vi "State Estimator.vi"(0 "Error In":errorcluster, 1 "State Estimate In":refnum<data-value>, 5 "Matrices":T6={"B"=[0.0, 0.0, 0.0, 0.0, 0.026179, 0.01, 0.0], "A"=[[1.0, 0.0, 0.0, 0.0, 0.0, 0.0, 0.01], [0.0, 1.0, 0.03, 0.0, 0.0, 0.01278, 0.0], [0.0, 0.0, 1.0, 0.0, 0.0, 0.025745, 0.0], [0.0, 0.0, 0.0, 1.0, 0.01, 0.0, 0.0], [0.0, 0.0, 0.0, 0.18884, 1.0, 0.13938, 0.0], [0.0, 0.0, 0.0, 0.0, 0.0, 1.0, 0.0], [0.0, 0.0, 0.0, 0.0, 0.0, 0.0, 1.0]], "C"=[[1.0, 0.0, 0.0, 0.0, 0.0, 0.0, 0.0], [0.0, 1.0, 0.0, 0.0, 0.0, 0.0, 0.0], [0.0, 0.0, 0.0, -13.87, 0.0, 4.7268, 0.0], [0.0, 0.0, 0.0, 0.0, 1.0, 0.0, 0.0], [0.0, 0.0, 0.0, 0.0, 0.0, 2.5745, 0.0], [0.0, 0.0, 0.0, 0.0, 0.0, 1.0, 0.0], [0.0, 0.0, 0.0, 0.0, 0.0, 0.0, 1.0]], "D"=[0.0, 0.0, -0.56285, 0.0, 0.0, 0.0, 0.0], "K"=[[0.61806, 0.0, 0.0, 0.0, 0.0, 0.0, 0.007236], [0.0, 0.64745, 1.9709e-05, 7.2294e-05, 0.0040091, 0.0015572, 0.0], [0.0, 0.60898, 2.0597e-05, 0.00027735, 0.0083707, 0.0032514, 0.0], [0.0, 2.3784e-05, 0.0, 0.0066165, 0.1014, 0.039387, 0.0], [0.0, 6.3434e-05, 0.0, 0.6191, 0.063823, 0.024791, 0.0], [0.0, 6.6011e-05, 0.0025018, 0.0011774, 0.29882, 0.11607, 0.0], [0.0010557, 0.0, 0.0, 0.0, 0.0, 0.0, 0.61803]], "Trajectory"=array601x3[1803 elements], "Init"=[0.0, 0.0, -0.56285, 0.0, 0.0, 0.0, 0.0]}, 7 "Configuration":T1={"Accelerometer Bias"={"X (m/s)"=0.0, "Y (m/s)"=0.0, "Z (m/s)"=0.0}, "Gyroscope Bias"={"X (m/s)"=0.0, "Y (m/s)"=0.0, "Z (m/s)"=0.0}, "Steering Motor Gear Ratio"=611.0, "Steering Pully Gear Ratio"=1.0, "Steering Encoder CPR"=500.0, "Steering Motor Max RPM"=4000.0, "Wheelbase (m)"=1.12, "Fork Angle (rad)"=1.3, "Balancing Controller"={"Kp (/s)"=1.0, "Kd (1)"=1.0}, "Max Allowed Steering Angle (rad)"=0.7, "Task Periods"={"Emergency Stop (us)"=10000, "IMU (us)"=10000, "Steering Motor Encoder (us)"=10000, "State Estimator (us)"=10000, "Balancing Controller (us)"=10000, "GNSS (us)"=10000, "Logging (us)"=50000, "Drive Motor (us)"=100000}, "Drive Motor Gear Ratio"=0.7, "lr"=0.0, "lf"=0.0, "lambda"=0.0, "k1"=0.0, "k2"=0.0, "e1_max"=0.0, "Ad_t"=0.0, "Bd_t"=0.0, "C_t"=0.0, "D_t"=0.0, "Wheel radius"=0.311}, 9 "Iteration":dbl, 11 "Measurement In":refnum<data-value>, 12 "Balancing controller In":refnum<data-value>) -> (4 "Error out":errorcluster, 15 "Measurement Out":refnum<data-value>)   [LabVIEW 2021]
uses:
  Measurements.ctl
  IMU/IMU Data.ctl
  Steering Motor Encoder/Steering Motor Encoder Data.ctl
  GNSS/GNSS Data.ctl
  Logging/Controller Data.ctl
  Drive Motor/Drive Motor Data.ctl
  Steering Motor/Steering Motor Data.ctl
  State Estimate.ctl
  Configuration/Configuration.ctl
panel:
  in  "Byte Stream File Refnum":refnum<file>
  out "Flag GPS":dbl
  out "State Estimate Out":refnum<data-value>
  out "data value":T2
  out "Input measurements":T5
  out "output cluster":T5 {"Y (m)" format="%#_10g"; "X (m)" format="%#_10g"}
  out "Balancing controller Out":refnum<data-value>
  in  "path in":path=path "libkalman_filter.so"
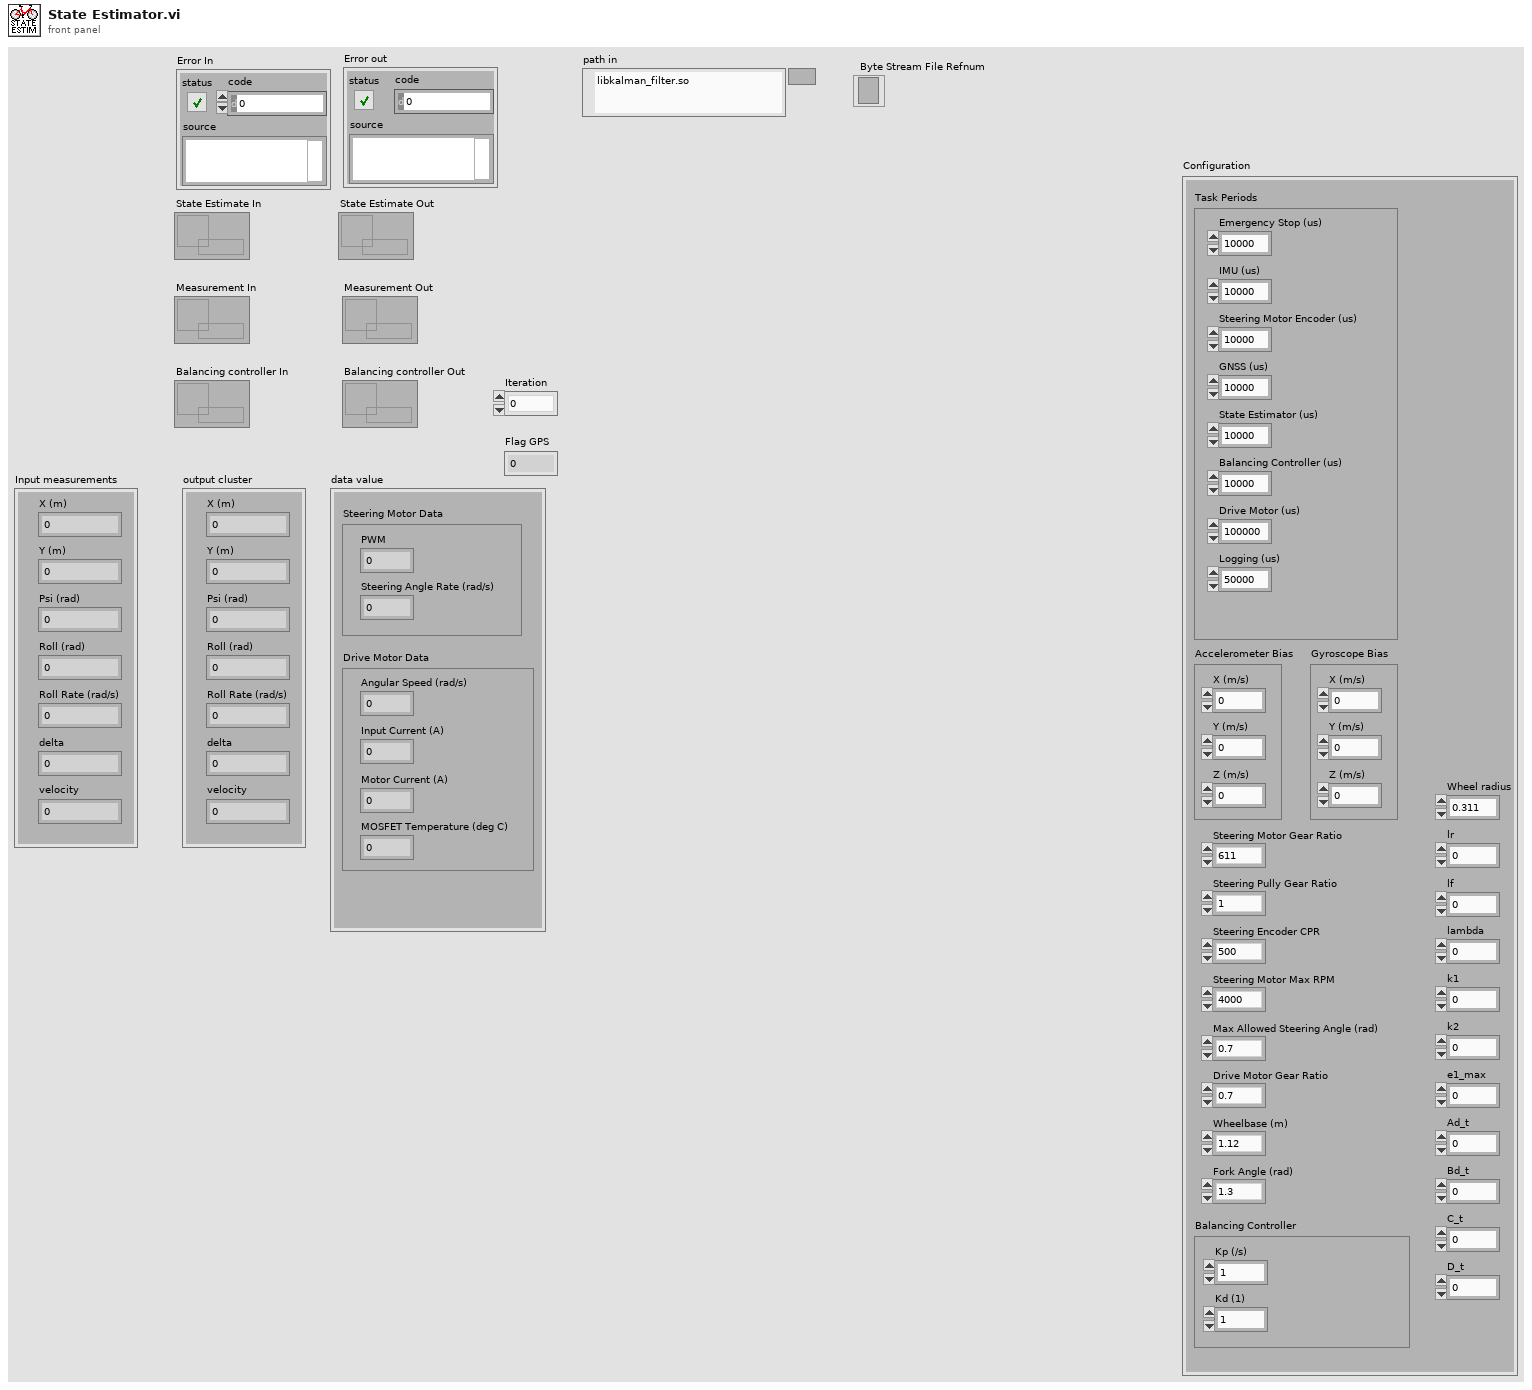
[diagram p1: front panel]
types:
  T1 = typedef "Configuration.ctl" = cluster{"Accelerometer Bias":cluster{"X (m/s)":dbl, "Y (m/s)":dbl, "Z (m/s)":dbl}, "Gyroscope Bias":cluster{"X (m/s)":dbl, "Y (m/s)":dbl, "Z (m/s)":dbl}, "Steering Motor Gear Ratio":dbl, "Steering Pully Gear Ratio":dbl, "Steering Encoder CPR":dbl, "Steering Motor Max RPM":dbl, "Wheelbase (m)":dbl, "Fork Angle (rad)":dbl, "Balancing Controller":cluster{"Kp (/s)":dbl, "Kd (1)":dbl}, "Max Allowed Steering Angle (rad)":dbl, "Task Periods":cluster{"Emergency Stop (us)":i64, "IMU (us)":i64, "Steering Motor Encoder (us)":i64, "State Estimator (us)":i64, "Balancing Controller (us)":i64, "GNSS (us)":i64, "Logging (us)":i64, "Drive Motor (us)":i64}, "Drive Motor Gear Ratio":dbl, "lr":dbl, "lf":dbl, "lambda":dbl, "k1":dbl, "k2":dbl, "e1_max":dbl, "Ad_t":dbl, "Bd_t":dbl, "C_t":dbl, "D_t":dbl, "Wheel radius":dbl}
  T2 = typedef "Controller Data.ctl" = cluster{"Drive Motor Data":T3, "Steering Motor Data":T4}
  T3 = typedef "Drive Motor Data.ctl" = cluster{"Angular Speed (rad/s)":dbl, "Input Current (A)":dbl, "Motor Current (A)":dbl, "MOSFET Temperature (deg C)":dbl}
  T4 = typedef "Steering Motor Data.ctl" = cluster{"PWM":dbl, "Steering Angle Rate (rad/s)":dbl}
  T5 = typedef "State Estimate.ctl" = cluster{"X (m)":dbl, "Y (m)":dbl, "Psi (rad)":dbl, "Roll (rad)":dbl, "Roll Rate (rad/s)":dbl, "delta":dbl, "velocity":dbl}
  T6 = cluster{"B":dbl[], "A":dbl[][], "C":dbl[][], "D":dbl[], "K":dbl[][], "Trajectory":dbl[][], "Init":dbl[]}
  T7 = typedef "Measurements.ctl" = cluster{"IMU Data":T8, "Steering Motor Encoder Data":T9, "GNSS Data":T10}
  T8 = typedef "IMU Data.ctl" = cluster{"Gyroscope":cluster{"X (rad/s)":dbl, "Y (rad/s)":dbl, "Z (rad/s)":dbl}, "Accelerometer":cluster{"X (m/s^2)":dbl, "Y (m/s^2)":dbl, "Z (m/s^2)":dbl}, "Flag IMU":dbl}
  T9 = typedef "Steering Motor Encoder Data.ctl" = cluster{"Encoder Position (counts)":i32, "Steering Angle (rad)":dbl, "Flag Steering Encoder":dbl}
  T10 = typedef "GNSS Data.ctl" = cluster{"Latitude (rad)":dbl, "Longitude (rad)":dbl, "Altitude (m)":dbl, "Speed (m/s)":dbl, "Heading (rad)":dbl, "Fix Quality":i32, "Number of Satellites":i32, "Latitude (deg)":dbl, "Longitude (deg)":dbl, "Flag GNSS":dbl}
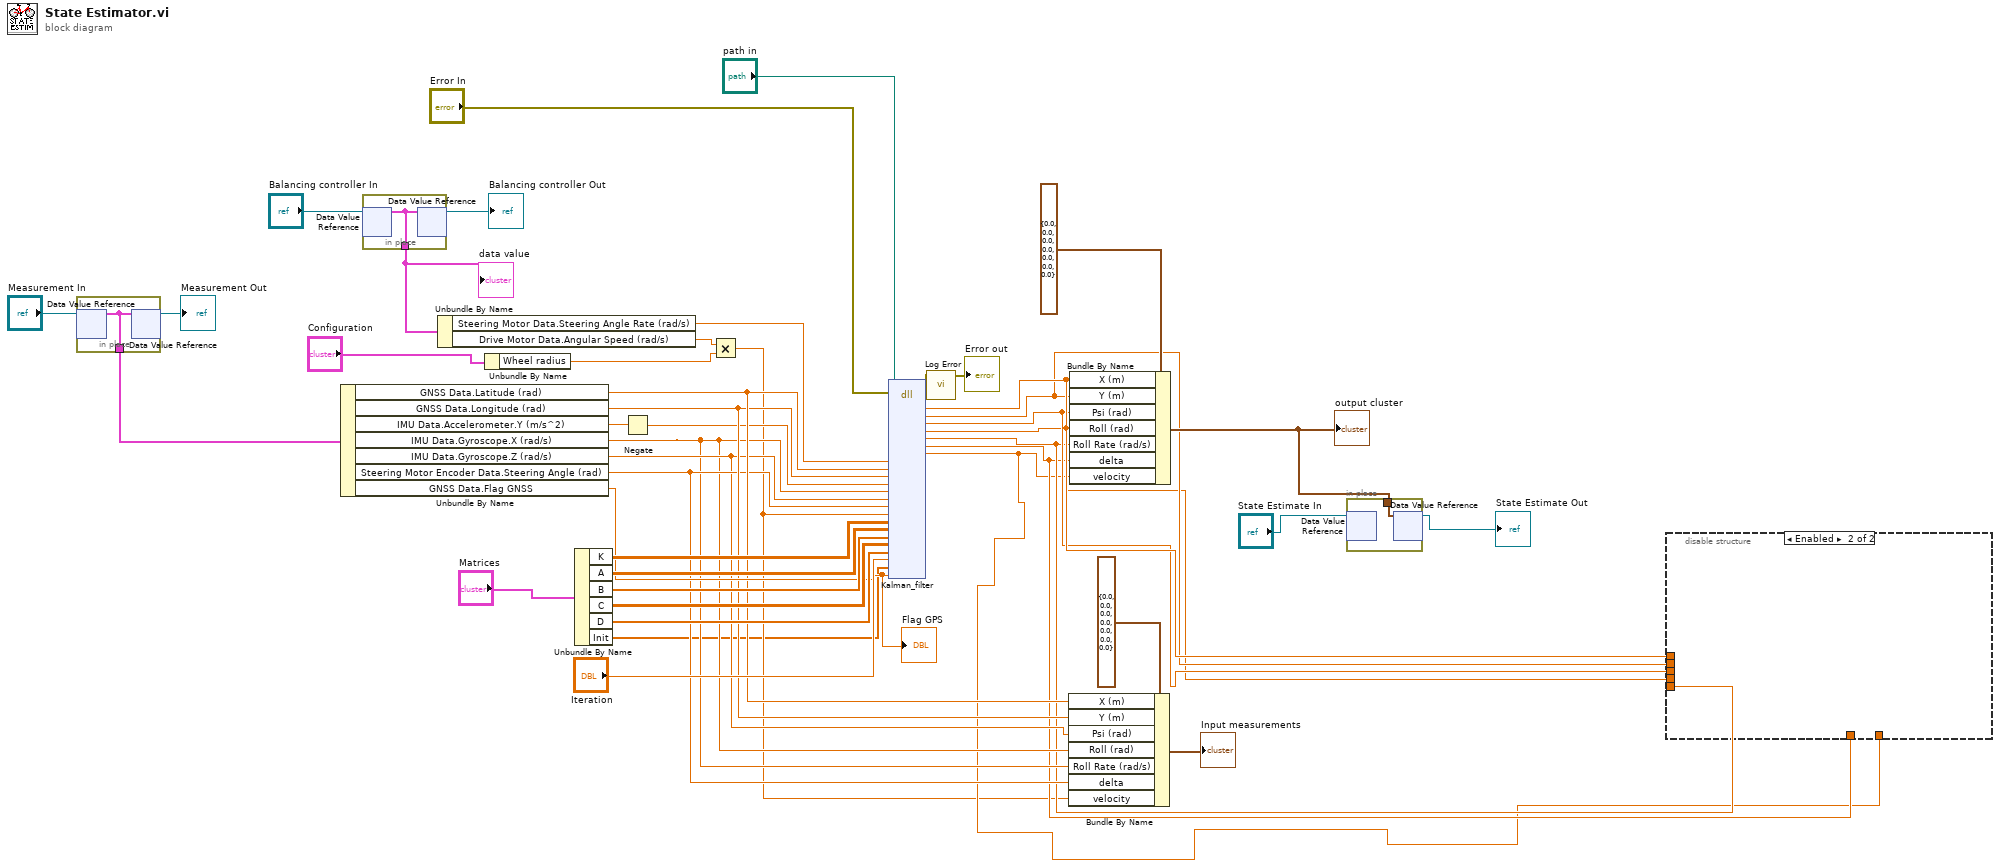
[diagram p0: block diagram]
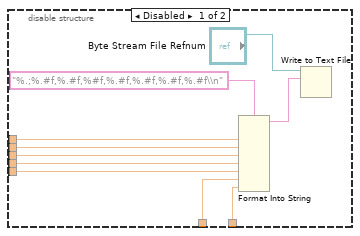
[diagram p2: hidden frame]
diagram:
  n1 = in-place {
    in-place-border: [w45] -> w35
    n2 = in-place-dvr #1("Measurement In") -> (w45:T7)  [unwired: 1 out]
    n3 = in-place-dvr #1(w45) -> (→"Measurement Out":refnum<data-value>)  [unwired: 1 out]
  }
  n4 = Unbundle By Name(w35) -> ("GNSS Data.Latitude (rad)"=w20:dbl, "GNSS Data.Longitude (rad)"=w19:dbl, "IMU Data.Accelerometer.Y (m/s^2)"=w16:dbl, "IMU Data.Gyroscope.X (rad/s)"=w12:dbl, "IMU Data.Gyroscope.Z (rad/s)"=w14:dbl, "Steering Motor Encoder Data.Steering Angle (rad)"=w17:dbl, "GNSS Data.Flag GNSS"=w21:dbl)
  "Flag GPS" <- w21
  n5 = in-place {
    in-place-border: [w46] -> w32
    n6 = in-place-dvr #2("Balancing controller In") -> (w46:T2)  [unwired: 1 out]
    n7 = in-place-dvr #2(w46) -> (→"Balancing controller Out":refnum<data-value>)  [unwired: 1 out]
  }
  "data value" <- w32
  n8 = Unbundle By Name(w32) -> ("Steering Motor Data.Steering Angle Rate (rad/s)"=w18:dbl, "Drive Motor Data.Angular Speed (rad/s)"=w4:dbl)
  n9 = Unbundle By Name("Configuration") -> ("Wheel radius"=w1:dbl)
  n10 = Unbundle By Name("Matrices") -> ("K"=w27:dbl[][], "A"=w26:dbl[][], "B"=w25:dbl[], "C"=w24:dbl[][], "D"=w23:dbl[], "Init"=w2:dbl[])
  n11 = Negate(x=w16) -> (-x=w15:dbl)
  n12 = Multiply(x=w4, y=w1) -> (x*y=w3:dbl)
  n13 = dll-call lib="libkalman_filter.so" fn="Kalman_filter"(path in="path in", error in="Error In", "dotdelta"=w18, "latitude"=w20, "longitude"=w19, "a_y"=w15, "w_x"=w12, "w_z"=w14, "delta_enc"=w17, "speed"=w3, "Kalman_Gain"=w27, "A_d"=w26, "B_d"=w25, "C"=w24, "D"=w23, "Reset"="Iteration", "init"=w2, "GPSflag"=w21) -> (error out=w28:errorcluster, "X"=w11:dbl, "Y"=w10:dbl, "Psi"=w9:dbl, "roll"=w8:dbl, "rollRate"=w7:dbl, "delta"=w6:dbl, "v"=w5:dbl)  [unwired: 25 in, 1 out]
  n14 = call "Log Error.vi"("Error In"=w28) -> ("Error Out"=→"Error out":errorcluster)  [unwired: 10 in]
  n15 = Bundle By Name(cluster=T5 {"X (m)"=0.0, "Y (m)"=0.0, "Psi (rad)"=0.0, "Roll (rad)"=0.0, "Roll Rate (rad/s)"=0.0, "delta"=0.0, "velocity"=0.0} ("State Estimate"), "X (m)"=w20, "Y (m)"=w19, "Psi (rad)"=w14, "Roll (rad)"=w12, "Roll Rate (rad/s)"=w12, "delta"=w17, "velocity"=w3) -> (→"Input measurements":T5)
  n16 = Bundle By Name(cluster=T5 {"X (m)"=0.0, "Y (m)"=0.0, "Psi (rad)"=0.0, "Roll (rad)"=0.0, "Roll Rate (rad/s)"=0.0, "delta"=0.0, "velocity"=0.0} ("State Estimate"), "X (m)"=w11, "Y (m)"=w10, "Psi (rad)"=w9, "Roll (rad)"=w8, "Roll Rate (rad/s)"=w7, "delta"=w6, "velocity"=w5) -> (w29:T5)
  "output cluster" <- w29
  n17 = in-place {
    in-place-border: w29 -> [w47]
    n18 = in-place-dvr #3("State Estimate In") -> ()  [unwired: 2 out]
    n19 = in-place-dvr #3(w47) -> (→"State Estimate Out":refnum<data-value>)  [unwired: 1 out]
  }
  n20 = disable-structure shown="Enabled" {
    disable-tunnel: w11 -> [w55 _]
    disable-tunnel: w10 -> [w54 _]
    disable-tunnel: w9 -> [w53 _]
    disable-tunnel: w8 -> [w52 _]
    disable-tunnel: w7 -> [w51 _]
    disable-tunnel: w6 -> [w50 _]
    disable-tunnel: w5 -> [w49 _]
    frame Disabled {
      n21 = Format Into String(format string="%.;%.#f,%.#f,%#f,%.#f,%.#f,%.#f,%.#f\\n", w55, w54, w53, w52, w51, w50, w49) -> (resulting string=w56:string)  [unwired: 2 in, 1 out]
      n22 = Write to Text File(file (use dialog)="Byte Stream File Refnum", text=w56) -> ()  [unwired: 2 in, 3 out]
    }
    frame Enabled {
    }
  }
